vi "iradon1 (SubVI).vi"(9 "N_det":dbl=40.0, 10 "N_rot":dbl=40.0, 11 "2-D Array of Real":dbl[][](array[numeric])) -> (3 "x/y":dbl[][](array[numeric]))   [LabVIEW 2018]
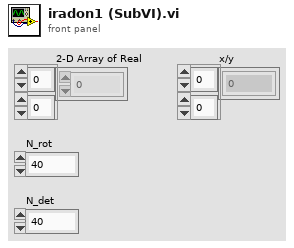
[diagram p1: front panel]
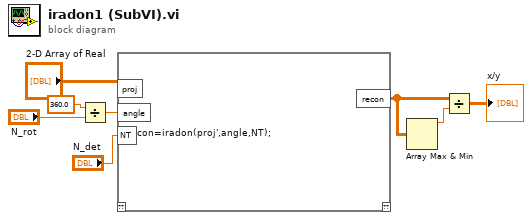
[diagram p0: block diagram]
diagram:
  n1 = Divide(x=360.0, y="N_rot") -> (x/y=w6:dbl)
  n2 = script code="recon=iradon(proj',angle,NT);"("proj"="2-D Array of Real", "angle"=w6, "NT"="N_det") -> ("recon"=w2:dbl[][])  [unwired: 1 in, 1 out]
  n3 = Array Max & Min(array=w2) -> (max value=w1:dbl)  [unwired: 3 out]
  n4 = Divide(x=w2, y=w1) -> (x/y=→"x/y":dbl[][])
